vi "Trajectory Reader.vi"() -> ()   [LabVIEW 2018]
uses:
  conversionTypeEnum.ctl
  <vilib>/Rock Robotics/WPI/ThirdParty/Phoenix-LabVIEW/Motor Controller/Get/CTRE_Phoenix_MotorController_GetClosedLoopData.vi
  <vilib>/Rock Robotics/WPI/ThirdParty/Phoenix-LabVIEW/Motor Controller/Get/CTRE_Phoenix_MotorController_GetSelectedSensorData.vi
panel:
  out "max(x,y)":i32
  out "Position":T1(graph)
  out "Position Error":i32(graph)
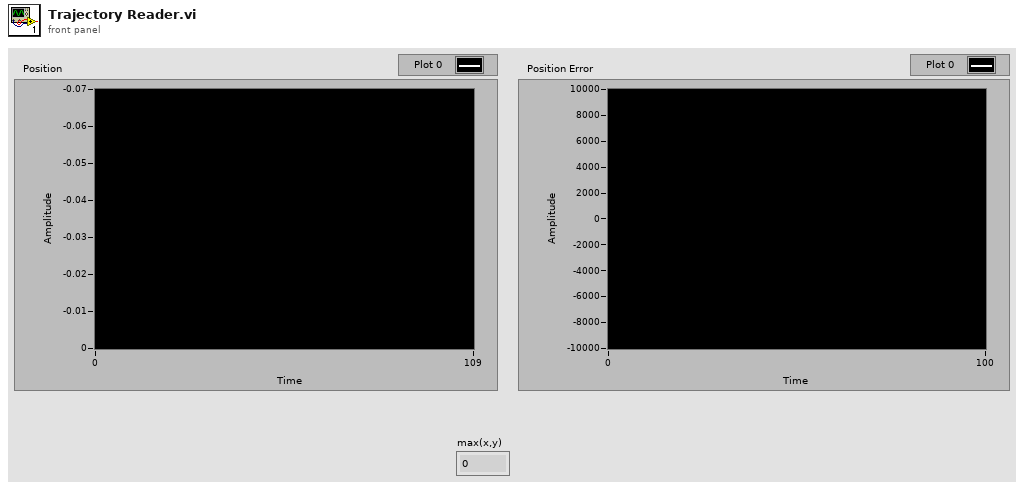
[diagram p1: front panel]
types:
  T1 = cluster{"Conversion Result":dbl, "Conversion Result":dbl}
  T2 = typedef "conversionTypeEnum.ctl" = enum16{"Sensor Units -> Inches", "Inches -> Sensor Units"}
  T3 = typedef "WPI_MotorControlDeviceRef.ctl" = cluster{"DeviceStatus":errorcluster, "Type":T4, "PWM":cluster{"PWM Channel":T5, "DeadBand":T6}, "CAN":cluster{"Device Number":u8, "SetOutput VI Ref":variant, "GetOutput VI Ref":variant, "Enable VI Ref":variant, "Disable VI Ref":variant, "Data":variant}, "Invert":bool, "DIO PWM":cluster{"PWM \"Enable\" Channel":T5, "DIOChannel":T7, "PWM Rate":dbl}}
  T4 = typedef "WPI_MotorControlType.ctl" = enum16{"PWM", "CAN", "DIO PWM"}
  T5 = typedef "FPGA_DIOPWMChannel.ctl" = enum8{"PWM 0", "PWM 1", "PWM 2", "PWM 3", "PWM 4", "PWM 5", "PWM 6", "PWM 7", "PWM 8", "PWM 9", "PWM MXP 0", "PWM MXP 1", "PWM MXP 2", "PWM MXP 3", "PWM MXP 4", "PWM MXP 5", "PWM MXP 6", "PWM MXP 7", "PWM MXP 8", "PWM MXP 9", "Invalid"}
  T6 = typedef "WPI_PWMDeadband.ctl" = cluster{"Name":string, "maxPositivePwm":i32, "minPositivePwm":i32, "centerPwm":i32, "maxNegativePwm":i32, "minNegativePwm":i32, "angularRange":u16}
  T7 = typedef "FPGA_DIOChannel.ctl" = enum8{"DIO 0", "DIO 1", "DIO 2", "DIO 3", "DIO 4", "DIO 5", "DIO 6", "DIO 7", "DIO 8", "DIO 9", "DIO MXP 0", "DIO MXP 1", "DIO MXP 2", "DIO MXP 3", "DIO MXP 4", "DIO MXP 5", "DIO MXP 6", "DIO MXP 7", "DIO MXP 8", "DIO MXP 9", "DIO MXP 10", "DIO MXP 11", "DIO MXP 12", "DIO MXP 13", "DIO MXP 14", "DIO MXP 15", "SPI Port CS1", "SPI Port CS2", "SPI Port CS3", "SPI Port MISO", "SPI Port MOSI", "Invalid"}
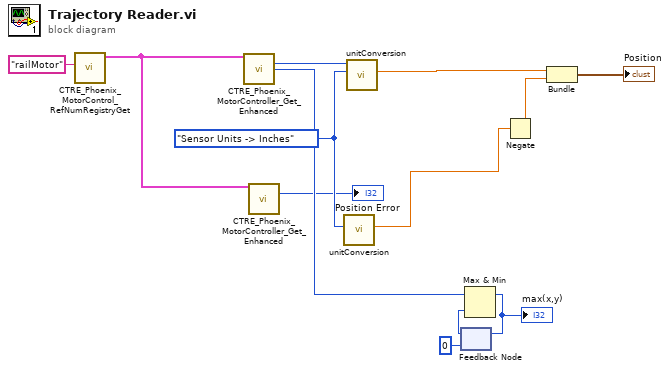
[diagram p0: block diagram]
diagram:
  w10 = conversionTypeEnum."Sensor Units -> Inches" ("Conversion Type")
  n1 = call <vilib>:"CTRE_Phoenix_MotorControl_RefNumRegistryGet.vi"("refnum name"="railMotor") -> ("PhoenixMotorControlDevRef"=w3:T3)  [unwired: 9 in, 1 out]
  n2 = call-poly <vilib>:"CTRE_Phoenix_MotorController_Get_Enhanced.vi"("PhoenixMotorControlDevRef"=w3) -> ("Position (Raw Sensor Units)"=w11:i32, "Velocity (Raw Sensor Units per 100 ms)"=w7:i32)  [unwired: 11 in, 2 out]
  n3 = call-poly <vilib>:"CTRE_Phoenix_MotorController_Get_Enhanced.vi"("PhoenixMotorControlDevRef"=w3) -> ("Closed-loop Error"=→"Position Error":i32)  [unwired: 9 in, 5 out]
  n4 = call "unitConversion.vi"("Conversion Type"=w10) -> ("Conversion Result"=w8:dbl)  [unwired: 10 in]
  n5 = call "unitConversion.vi"("Conversion Type"=w10, "Units to Convert"=w11) -> ("Conversion Result"=w9:dbl)  [unwired: 9 in]
  n6 = feedback #1(0) -> (w5:i32)
  n7 = Max & Min(x=w7, y=w5) -> (max(x,y)=w6:i32)  [unwired: 1 out]
  "max(x,y)" <- w6
  n8 = feedback-in #1(w6) -> ()
  n9 = Negate(x=w8) -> (-x=w4:dbl)
  n10 = Bundle("Conversion Result"=w9, w4) -> (→"Position":cluster{"Conversion Result":dbl, dbl})  [unwired: 1 in]
